vi "GetImpairReports.vi"(8 "error in (no error)":errorcluster, 11 "SineModelPlugin in":refnum<class "SineModelPlugin.lvclass">) -> (0 "error out":errorcluster, 3 "SineModelPlugin out":refnum<class "SineModelPlugin.lvclass">)   [LabVIEW 2017, in "PmuImpairPlugins.lvlib" / "SineModelPlugin.lvclass"]
uses:
  SineModelPlugin.lvclass
  C:/dev/Work/PARTF/Modules/PmuImpairPlugins/PmuImpairPluginBase_class/PmuImpairPluginBase.lvclass
  PmuImpairPluginBase_class/PmuImpairPluginBase.lvclass/PmuImpairPluginBase.ctl
  EventPlugins/EventPluginBaseClass/TypeDefs/clEvtReport.ctl
  PmuImpairPluginBase_class/Accessors/Read BusNumber.vi
  PmuImpairPluginBase_class/Accessors/Read clImpairConfig.vi
  PmuImpairPluginBase_class/Accessors/Read dblImpairParams.vi
  EventPlugins/EventPluginBaseClass/EventPluginBaseClass.lvclass
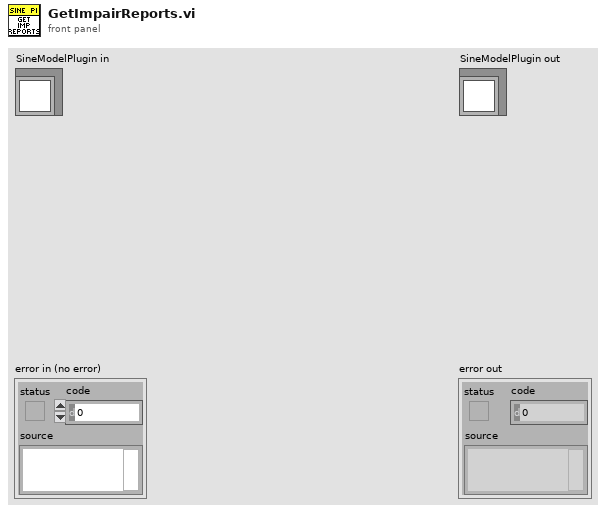
[diagram p1: front panel]
types:
  T1 = typedef "EventPlugins.lvlib/EventPluginBaseClass.lvclass/clEvtReport.ctl" = cluster{"Timestamp":dbl, "Synx":cdb[], "Freq":dbl, "ROCOF":dbl, "ID":i16}
  T2 = typedef "PmuImpairPlugins.lvlib/PmuImpairPluginBase.lvclass/clImpairConfig.ctl" = cluster{"FilterType":string, "bPosSeq":bool}
  T3 = typedef "EventPlugins.lvlib/EventPluginBaseClass.lvclass/clEvtReportArray.ctl" = T1[]
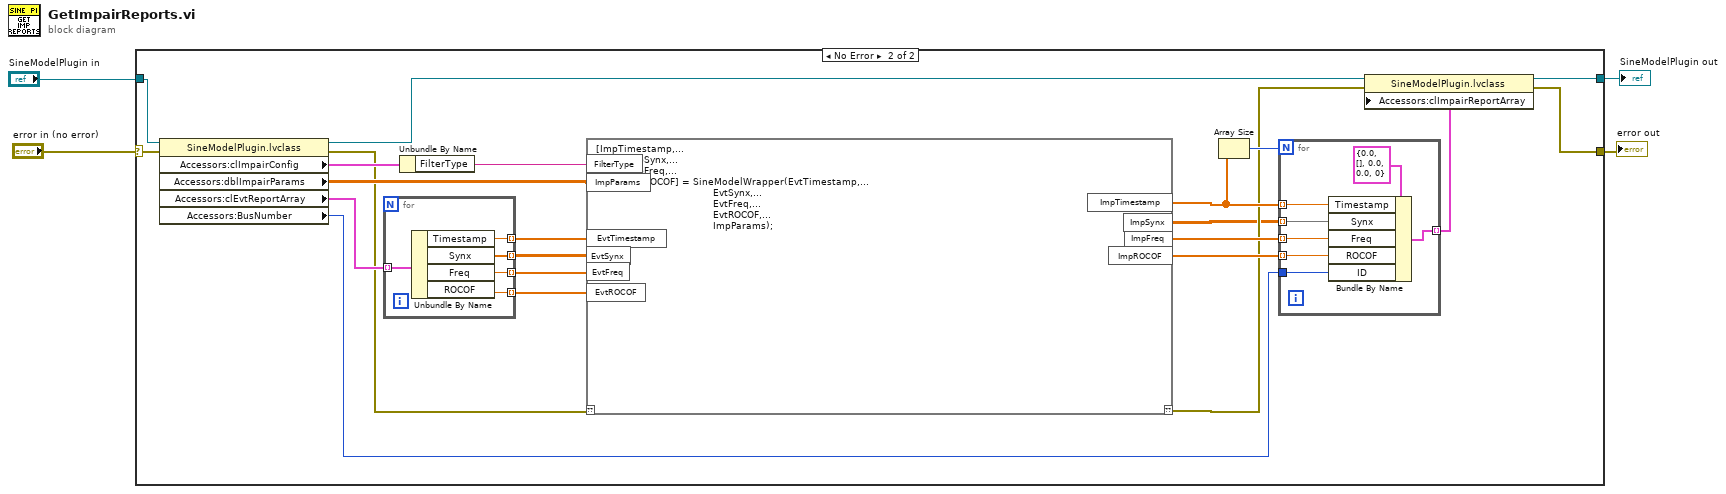
[diagram p0: block diagram]
diagram:
  n1 = case shown="No Error" "error in (no error)" {
    selector: "error in (no error)" -> [w6 w23]
    tunnel: [w5 w26] -> w4
    tunnel: "SineModelPlugin in" -> [w5 w24]
    tunnel: [w6 w25] -> w1
    frame Error {
    }
    frame No Error {
      n2 = property class="SineModelPlugin.lvclass"(reference=w24, error in=w23) -> (reference out=w22:refnum<class "SineModelPlugin.lvclass">, error out=w8:errorcluster, "Accessors:clImpairConfig"=w16:T2, "Accessors:dblImpairParams"=w17:dbl[][], "Accessors:clEvtReportArray"=w14:T3, "Accessors:BusNumber"=w7:u8)
      n3 = for {
        tunnel: w14 -> [w33] mode=indexing
        tunnel: [w32] -> w13 mode=indexing
        tunnel: [w31] -> w12 mode=indexing
        tunnel: [w30] -> w11 mode=indexing
        tunnel: [w29] -> w10 mode=indexing
        n4 = Unbundle By Name(w33) -> ("Timestamp"=w32:dbl, "Synx"=w31:cdb[], "Freq"=w30:dbl, "ROCOF"=w29:dbl)
      }
      n5 = Unbundle By Name(w16) -> ("FilterType"=w15:string)
      n6 = script code="[ImpTimestamp,...\n          ImpSynx,...\n          ImpFreq,...\n          ImpROCOF] = SineModelWrapper(EvtTimestamp,...\n                                       EvtSynx,...\n                                       EvtFreq,...\n                                       EvtROCOF,...\n                                       ImpParams);"("??"=w8, "FilterType"=w15, "ImpParams"=w17, "EvtTimestamp"=w13, "EvtSynx"=w12, "EvtFreq"=w11, "EvtROCOF"=w10) -> ("??"=w19:errorcluster, "ImpTimestamp"=w21:dbl[], "ImpFreq"=w28:dbl[], "ImpROCOF"=w27:dbl[], "ImpSynx"=w18:cdb[][])
      n7 = Array Size(array=w21) -> (size(s)=w20:i32)
      n8 = for {
        N: w20 -> [_]
        tunnel: w21 -> [w40] mode=indexing
        tunnel: w28 -> [w39] mode=indexing
        tunnel: w27 -> [w38] mode=indexing
        tunnel: w18 -> [w37] mode=indexing
        tunnel: [w35] -> w9 mode=indexing
        tunnel: w7 -> [w34]
        n9 = Bundle By Name(cluster=T1 {"Timestamp"=0.0, "Synx"=[], "Freq"=0.0, "ROCOF"=0.0, "ID"=0} ("clEvtReport"), "Timestamp"=w40, "Synx"=w37, "Freq"=w39, "ROCOF"=w38, "ID"=w34) -> (w35:T1)
      }
      n10 = property class="SineModelPlugin.lvclass"(reference=w22, error in=w19, "Accessors:clImpairReportArray"=w9) -> (reference out=w26:refnum<class "SineModelPlugin.lvclass">, error out=w25:errorcluster)
    }
  }
  "error out" <- w1
  "SineModelPlugin out" <- w4
